vi "Dashboard Main - Copy.vi"() -> ()   [LabVIEW 2011]
panel:
  out "TARGET AQUIRED":bool
  out "FAILSAFE!":bool
  out "Right":T1(plugin-control)
  out "Left":T1(plugin-control)
  in  "Tab Control":enum32{"Operator", "Diagnotics"}(tab)
  out "Shooter RPM":dbl(knob) scale=0.0..4000.0
  out "Limit Right":bool
  out "Limit Left":bool
  out "Turret Postition":dbl(knob) scale=240.0..-60.0
  out "Home":bool
  out "1":bool
  out "2":bool
  out "3":bool
  out "Bridge Balance":bool
  out "Intake Reverse":bool
  out "Intake Foward":bool
  out "High Gear":bool
  out "Low Gear":bool
  out "Robot IP Address":string
  out "Battery Voltage":dbl(slide) scale=8.0..14.0
  out "Distance From Target":dbl
  in  "Distance adjust":dbl
  in  "Left camera adjust":dbl
  in  "Right camera adjust":dbl
  out "Turret Enc":dbl
  out "Compass":dbl(knob) scale=0.0..-180.0
  out "Shooter Ready":bool
  out "Right Drive":dbl
  out "Left Drive":dbl
  out "Gyro":dbl(knob) scale=-180.0..180.0
  out "Primed":bool
  out "Upper Belt":bool
  out "Lower Belt":bool
  out "Entrance":bool
  in  "Video Enable":bool=TRUE
  in  "LED Color":enum32{"RED", "BLUE", "PURPLE"}(radio)
  out "FIRE!":bool
  out "Dashboard Datatype Warning":string="Warning: The Dashboard Datatype used by the robot project and this dashboard do not match.\nSee diagram for more details."
  # "Ball Count"
  # "Communications"
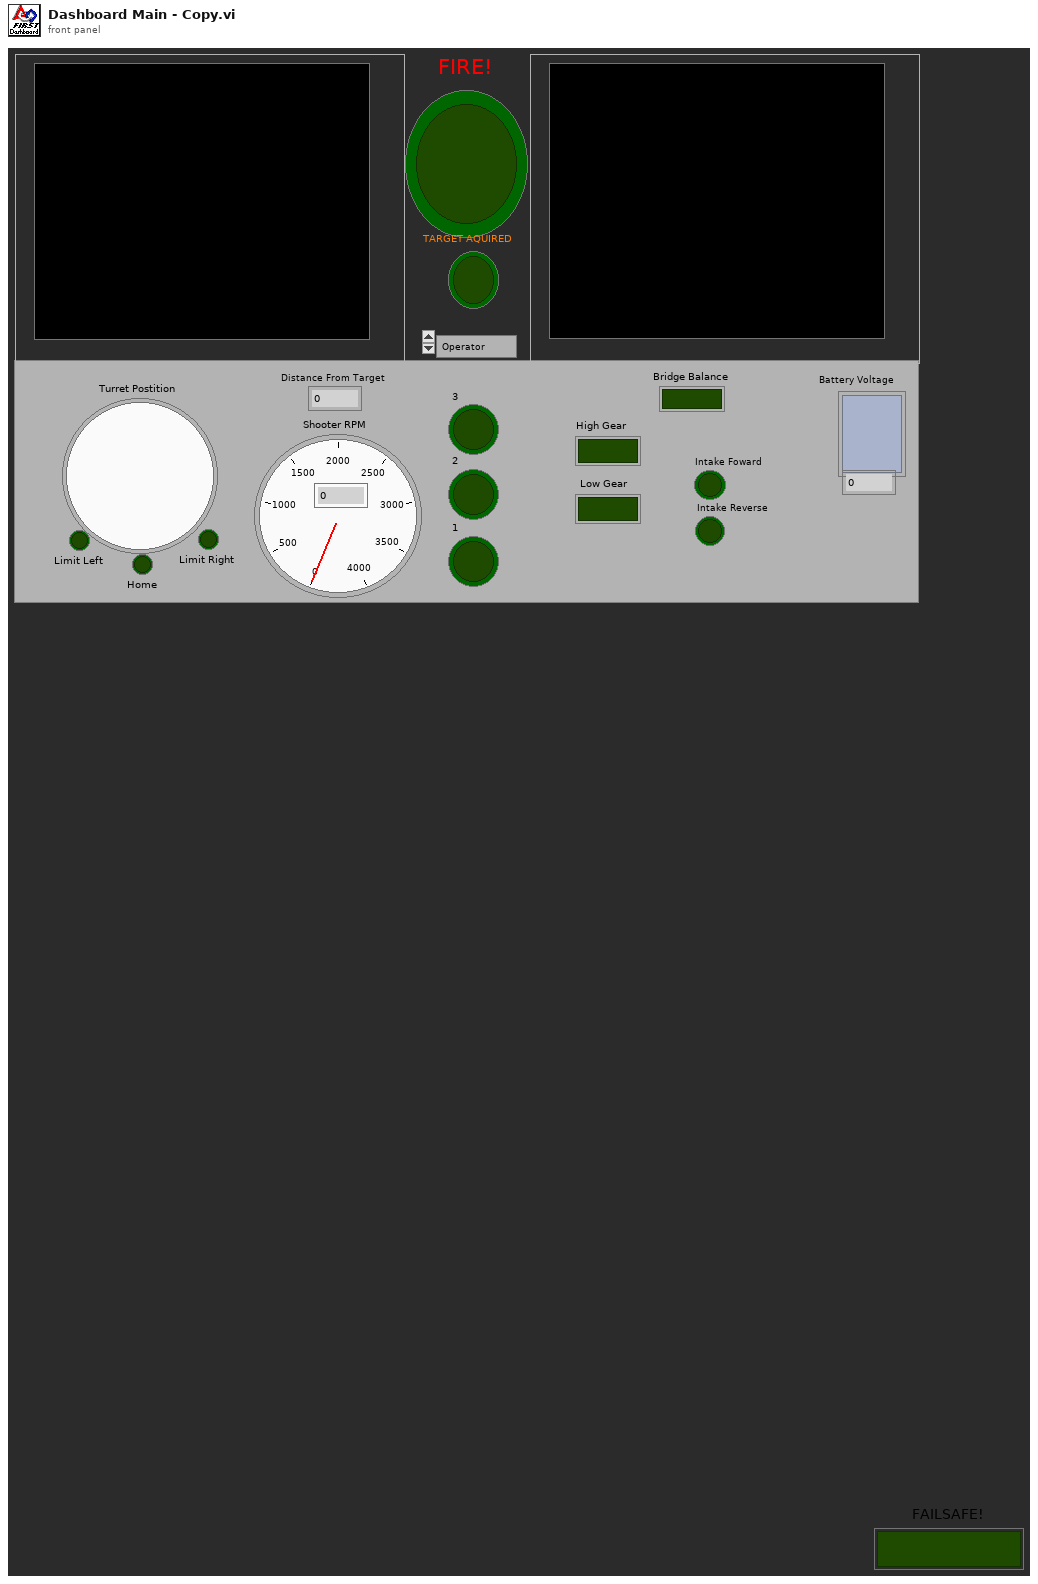
[diagram p1: front panel]
types:
  T1 = typedef "IMAQ Image.ctl" = refnum<image>
  T2 = cluster{"Home":bool, "Distance From Target":dbl, "Ball Count":dbl, "Gear":u16, "Shooter RMP":dbl, "Target Acuired":bool, "FIRE":bool, "Intake Motor direction":dbl, "FailSafe":bool}
  T3 = cluster{"Distance From Target":dbl, "Bridge Balance":bool, "Entrance":bool, "Lower Belt":bool, "Upper Belt":bool, "Primed":bool, "Turret Postition":dbl, "Gyro":dbl, "Left Drive":dbl, "Right Drive":dbl, "Home":bool, "Limit Left":dbl, "Limit Right":dbl, "Shooter Ready":bool, "Compass":dbl, "Turret Enc":dbl, "Ball Count":dbl, "Intake":dbl}
  T4 = typedef "Image Type" = u32
  T5 = cluster{"Competition mode":bool, "Robot Link":bool, "Autonomous":bool, "Enabled":bool, "E-Stop":bool}
  T6 = cluster{"Boolean array[0]":bool, "Boolean array[1]":bool, "Boolean array[2]":bool, "Boolean array[3]":bool, "Boolean array[4]":bool, "Boolean array[5]":bool, "Boolean array[6]":bool, "Boolean array[7]":bool, "Boolean array[8]":bool}
  T7 = typedef "LVRectTypeDef.ctl" = cluster{"left":i16, "top":i16, "right":i16, "bottom":i16}
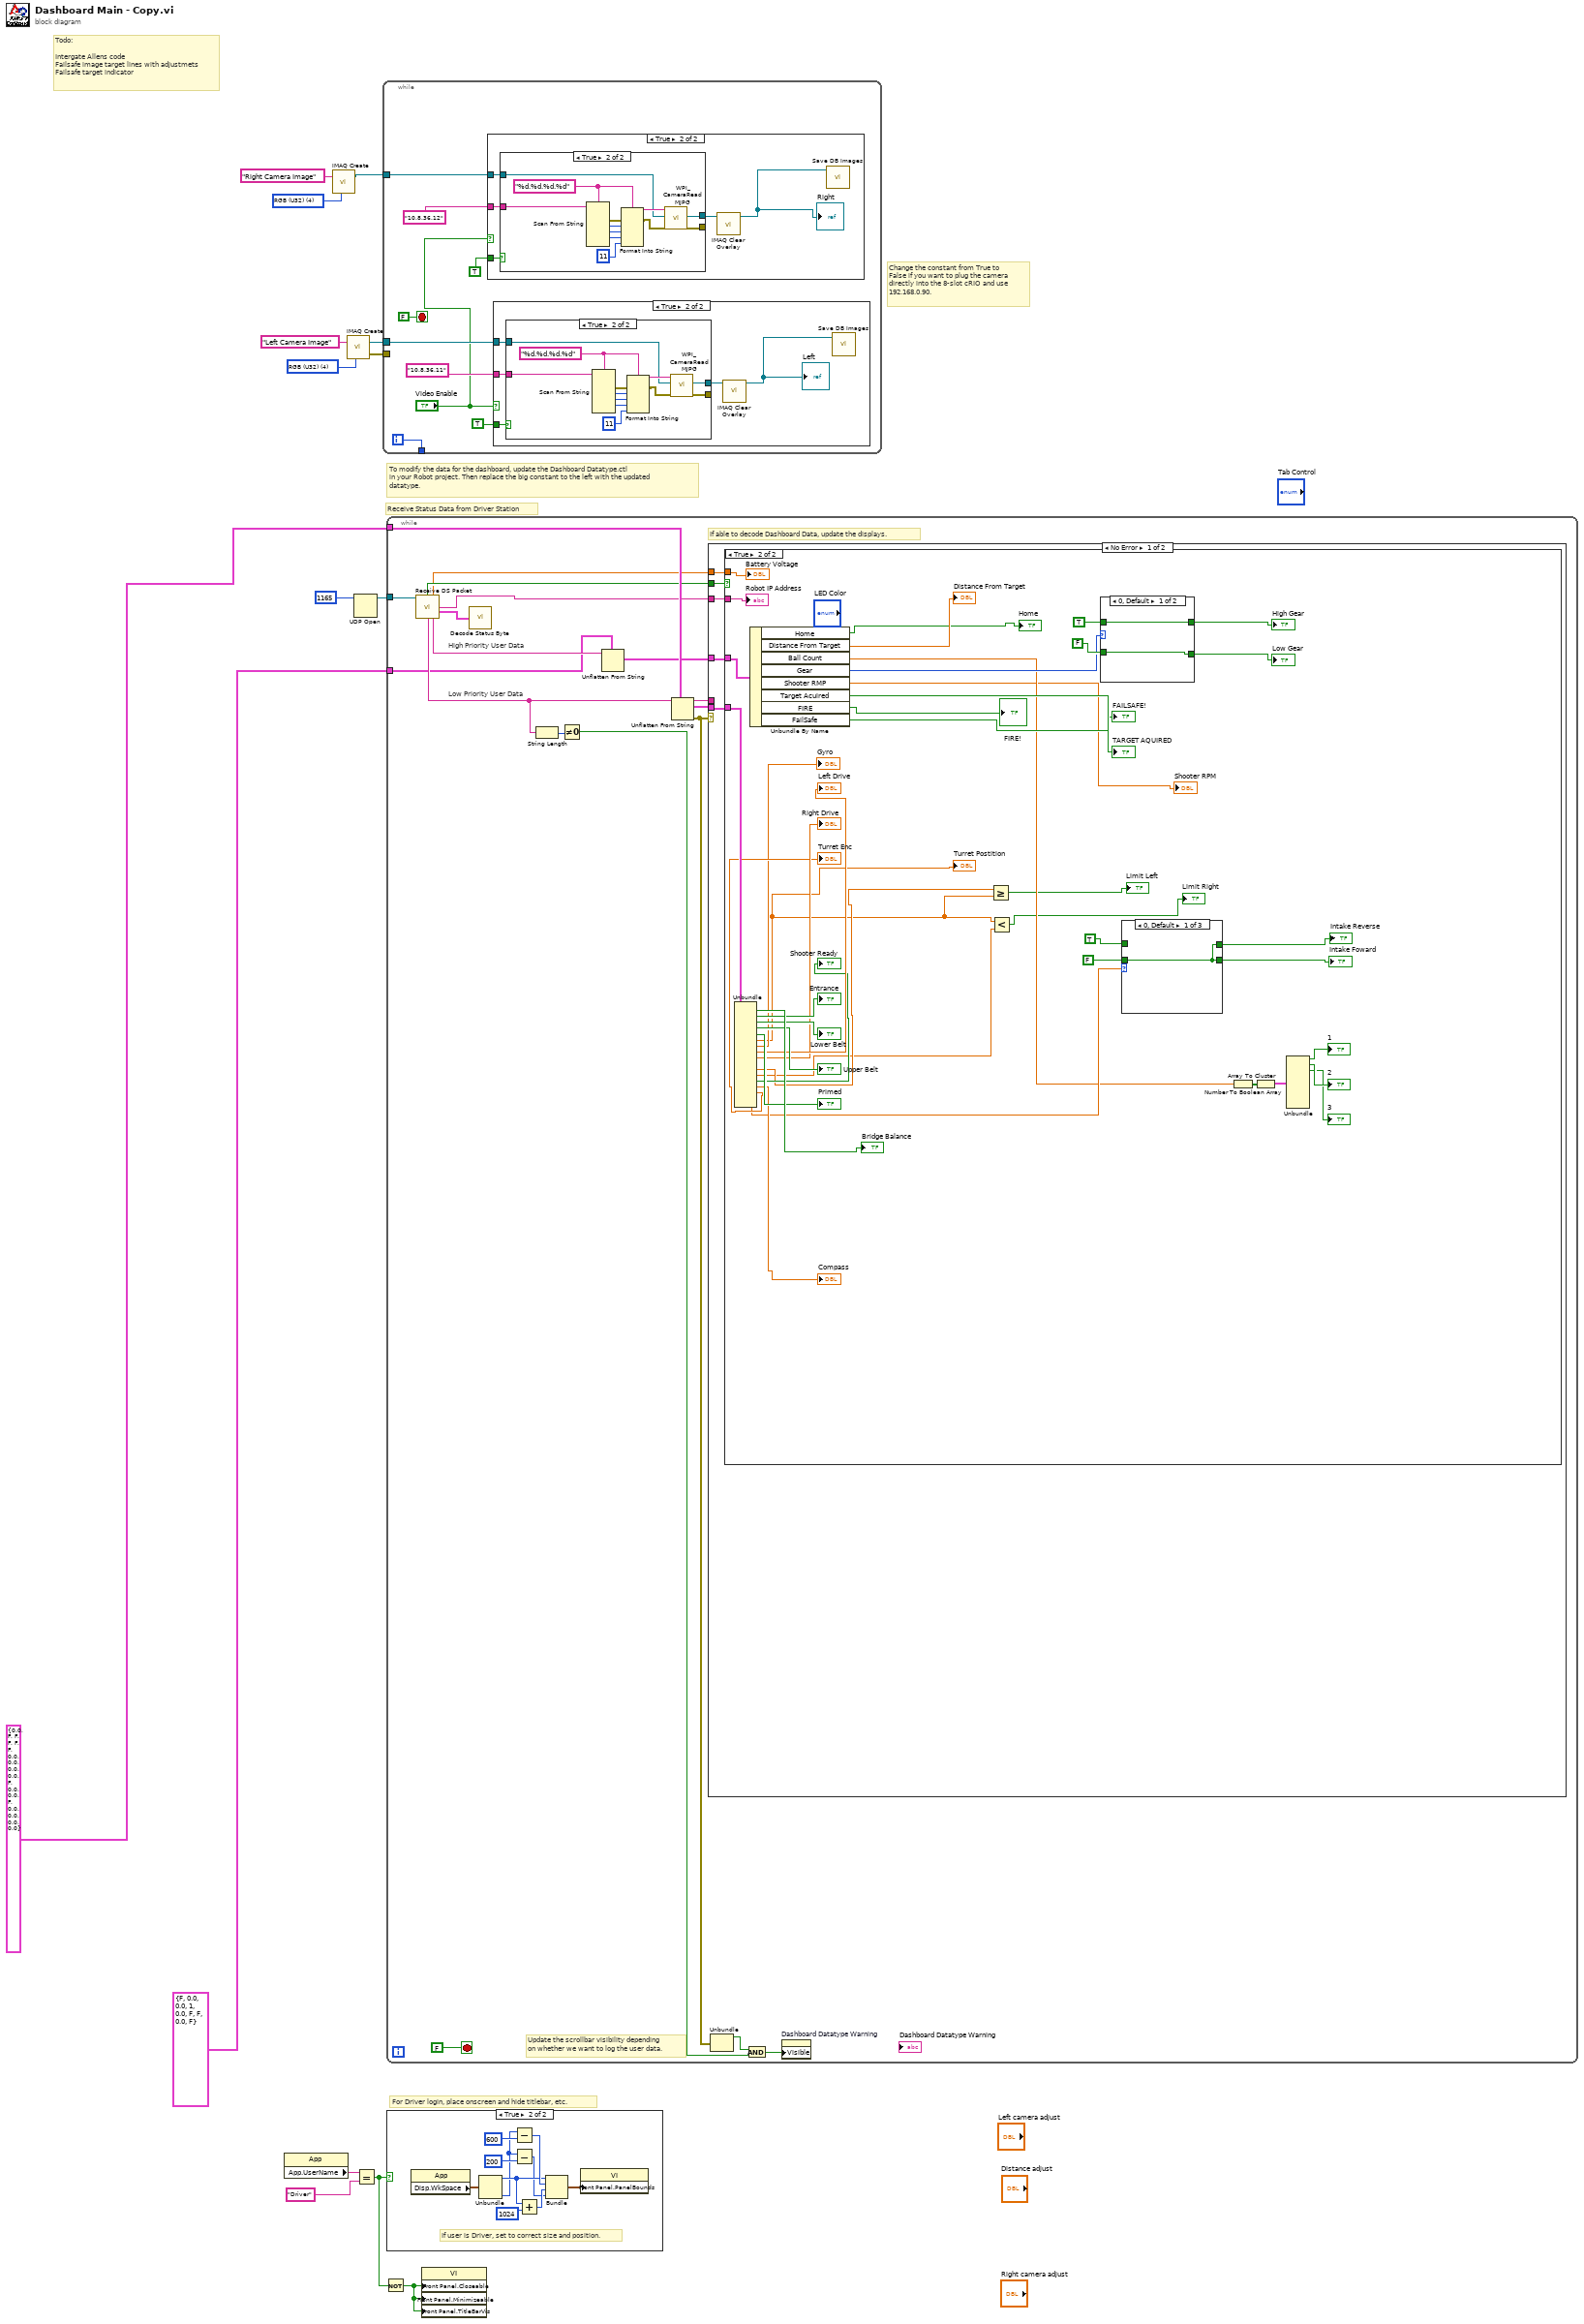
[diagram p0: block diagram]
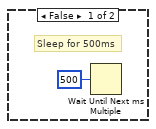
[diagram p8: hidden frame]
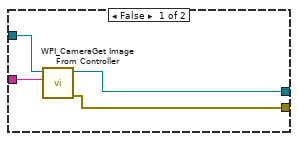
[diagram p9: hidden frame]
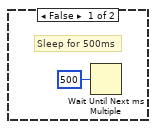
[diagram p10: hidden frame]
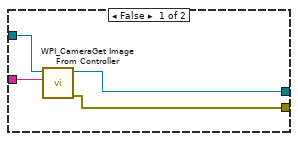
[diagram p11: hidden frame]
diagram:
  w5 = T4 4 items=["Grayscale (U8)", "Grayscale (I16)", "Grayscale (SGL)", "Complex (CSG)", "RGB (U32)", "HSL (U32)", "RGB (U64)"] ("Image Type")
  w13 = T4 4 items=["Grayscale (U8)", "Grayscale (I16)", "Grayscale (SGL)", "Complex (CSG)", "RGB (U32)", "HSL (U32)", "RGB (U64)"] ("Image Type")
  # "Todo: \n\nIntergate Allens code\nFailsafe image target lines with adjustmets\nFailsafe target indicator"
  # "Change the constant from True to\nFalse if you want to plug the camera\ndirectly into the 8-slot cRIO and use\n192.168.0.90."
  # "For Driver login, place onscreen and hide titlebar, etc."
  # "To modify the data for the dashboard, update the Dashboard Datatype.ctl\nin your Robot project. Then replace the big constant to the left with the updated\ndatatype."
  # "Receive Status Data from Driver Station"
  n1 = property class="App"() -> ("App.UserName"=w8:string)  [unwired: 2 in, 2 out]
  n2 = call "IMAQ Create"("Image Name"="Right Camera Image", "Image Type"=w5) -> ("New Image"=w3:T1)  [unwired: 2 in, 2 out]
  n3 = call "IMAQ Create"("Image Name"="Left Camera Image", "Image Type"=w13) -> ("New Image"=w11:T1, "error out"=w10:errorcluster)  [unwired: 2 in, 1 out]
  n4 = UDP Open(11:u16 1165 ("port")) -> (port=w14:refnum<k16>)  [unwired: 2 in, 4 out]
  n5 = Equal?(x=w8, y="Driver") -> (x = y?=w7:bool)
  n6 = while {
    tunnel: w11 -> [w23]
    tunnel: w10 -> [_]
    tunnel: [w21] -> _
    tunnel: w3 -> [w17]
    i -> [w21]
    stop <- FALSE stop-if-true
    n7 = case shown="True" "Video Enable" {
      tunnel: "10.8.36.12" ("input string") -> [_ w30]
      tunnel: w17 -> [_ w29]
      tunnel: TRUE -> [_ w27]
      frame False {
        # "Sleep for 500ms"
        n8 = Wait Until Next ms Multiple(millisecond multiple=u32 500) -> ()  [unwired: 1 out]
      }
      frame True {
        n9 = case shown="True" w27 {
          tunnel: w29 -> [w33 w40]
          tunnel: [w31 w38] -> _
          tunnel: [w32 w39] -> w28
          tunnel: w30 -> [w34 w43]
          frame False {
            n10 = call <vilib>:"WPI_CameraGet Image From Controller.vi"("Controller Address"=w34, "Image"=w33) -> ("error out"=w31:errorcluster, "Image Out"=w32:T1)  [unwired: 2 in, 6 out]
          }
          frame True {
            w35 = "%d.%d.%d.%d" ("format string")
            n11 = Scan From String(format string=w35, input string=w43) -> (error out=w42:errorcluster, output 1=w44:i32, output 2=w45:i32, output 3=w46:i32)  [unwired: 2 in, 7 out]
            n12 = Format Into String(format string=w35, error in=w42, w44, w45, w46, 11 ("IP Suffix:")) -> (resulting string=w41:string, error out=w37:errorcluster)  [unwired: 1 in]
            n13 = call <vilib>:"WPI_CameraRead MJPG.vi"("error in"=w37, "Image"=w40, "address"=w41) -> ("error out"=w38:errorcluster, "Image Out"=w39:T1)  [unwired: 7 in]
          }
        }
        n14 = call "IMAQ Clear Overlay"("Image"=w28) -> ("Image Out"=w26:T1)  [unwired: 2 in, 8 out]
        "Right" <- w26
        n15 = call "Save DB Images.vi"("Image"=w26) -> ()  [unwired: 2 in, 1 out]
      }
    }
    n16 = case shown="True" "Video Enable" {
      tunnel: "10.8.36.11" ("input string") -> [_ w52]
      tunnel: w23 -> [_ w51]
      tunnel: TRUE -> [_ w49]
      frame False {
        # "Sleep for 500ms"
        n17 = Wait Until Next ms Multiple(millisecond multiple=u32 500) -> ()  [unwired: 1 out]
      }
      frame True {
        n18 = case shown="True" w49 {
          tunnel: w51 -> [w55 w62]
          tunnel: [w53 w60] -> _
          tunnel: [w54 w61] -> w50
          tunnel: w52 -> [w56 w65]
          frame False {
            n19 = call <vilib>:"WPI_CameraGet Image From Controller.vi"("Controller Address"=w56, "Image"=w55) -> ("error out"=w53:errorcluster, "Image Out"=w54:T1)  [unwired: 2 in, 6 out]
          }
          frame True {
            w57 = "%d.%d.%d.%d" ("format string")
            n20 = Scan From String(format string=w57, input string=w65) -> (error out=w64:errorcluster, output 1=w66:i32, output 2=w67:i32, output 3=w68:i32)  [unwired: 2 in, 7 out]
            n21 = Format Into String(format string=w57, error in=w64, w66, w67, w68, 11 ("IP Suffix:")) -> (resulting string=w63:string, error out=w59:errorcluster)  [unwired: 1 in]
            n22 = call <vilib>:"WPI_CameraRead MJPG.vi"("error in"=w59, "Image"=w62, "address"=w63) -> ("error out"=w60:errorcluster, "Image Out"=w61:T1)  [unwired: 7 in]
          }
        }
        n23 = call "IMAQ Clear Overlay"("Image"=w50) -> ("Image Out"=w48:T1)  [unwired: 2 in, 8 out]
        "Left" <- w48
        n24 = call "Save DB Images.vi"("Image"=w48) -> ()  [unwired: 2 in, 1 out]
      }
    }
  }
  n25 = Not(x=w7) -> (.not. x?=w6:bool)
  n26 = while {
    tunnel: w14 -> [w84]
    tunnel: T3 {"Distance From Target"=0.0, "Bridge Balance"=FALSE, "Entrance"=FALSE, "Lower Belt"=FALSE, "Upper Belt"=FALSE, "Primed"=FALSE, "Turret Postition"=0.0, "Gyro"=0.0, "Left Drive"=0.0, "Right Drive"=0.0, "Home"=FALSE, "Limit Left"=0.0, "Limit Right"=0.0, "Shooter Ready"=FALSE, "Compass"=0.0, "Turret Enc"=0.0, "Ball Count"=0.0, "Intake"=0.0} ("Dashboard Data") -> [w83]
    tunnel: T2 {"Home"=FALSE, "Distance From Target"=0.0, "Ball Count"=0.0, "Gear"=1, "Shooter RMP"=0.0, "Target Acuired"=FALSE, "FIRE"=FALSE, "Intake Motor direction"=0.0, "FailSafe"=FALSE} ("HiPri") -> [w70]
    stop <- FALSE stop-if-true
    # "High Priority User Data"
    # "Low Priority User Data"
    # "Update the scrollbar visibility depending\non whether we want to log the user data."
    # "If able to decode Dashboard Data, update the displays."
    n27 = call "Receive DS Packet.vi"("Recv Socket"=w84) -> ("New Dashboard Data"=w80:bool, "Battery"=w72:sgl, "Robot IP Address"=w71:string, "Status"=w85:T5, "Low Priority User Data"=w74:string, "High Priority User Data"=w73:string)  [unwired: 1 in, 8 out]
    n28 = call "Decode Status Byte.vi"("Status Byte"=w85) -> ()  [unwired: 2 out]
    n29 = String Length(string=w74) -> (length=w75:i32)
    n30 = Not Equal To 0?(x=w75) -> (x != 0?=w78:bool)
    n31 = Unflatten From String(type=w70, binary string=w73) -> (value=w69:T2)  [unwired: 1 in, 4 out]
    n32 = Unflatten From String(type=w83, binary string=w74) -> (rest of the binary string=w76:string, value=w82:T3, error out=w81:errorcluster)  [unwired: 1 in, 2 out]
    n33 = case shown="No Error" w81 {
      tunnel: w82 -> [w91 _]
      tunnel: w80 -> [w90 _]
      tunnel: w76 -> [_ _]
      tunnel: w72 -> [w89 _]
      tunnel: w71 -> [w88 _]
      tunnel: w69 -> [w87 _]
      frame No Error {
        n34 = case shown="True" w90 {
          tunnel: w91 -> [_ w133]
          tunnel: w89 -> [_ w132]
          tunnel: w88 -> [_ w131]
          tunnel: w87 -> [_ w103]
          frame False {
            # "Don't update if the robot hasn't sent new data"
          }
          frame True {
            n35 = Unbundle(w133) -> ("Bridge Balance"=→"Bridge Balance":bool, "Entrance"=→"Entrance":bool, "Lower Belt"=→"Lower Belt":bool, "Upper Belt"=→"Upper Belt":bool, "Primed"=→"Primed":bool, "Turret Postition"=w92:dbl, "Gyro"=→"Gyro":dbl, "Left Drive"=→"Left Drive":dbl, "Right Drive"=→"Right Drive":dbl, "Limit Left"=w105:dbl, "Limit Right"=w104:dbl, "Shooter Ready"=→"Shooter Ready":bool, "Compass"=→"Compass":dbl, "Turret Enc"=→"Turret Enc":dbl, "Intake"=w107:dbl)  [unwired: 3 out]
            "Turret Postition" <- w92
            n36 = Unbundle By Name(w103) -> ("Home"=→"Home":bool, "Distance From Target"=→"Distance From Target":dbl, "Ball Count"=w98:dbl, "Gear"=w101:u16, "Shooter RMP"=→"Shooter RPM":dbl, "Target Acuired"=→"TARGET AQUIRED":bool, "FIRE"=→"FIRE!":bool, "FailSafe"=→"FAILSAFE!":bool)
            n37 = Greater Or Equal?(x=w105, y=w92) -> (x >= y?=→"Limit Left":bool)
            n38 = Less?(x=w92, y=w104) -> (x < y?=→"Limit Right":bool)
            n39 = case shown="0, Default" w101 {
              tunnel: TRUE -> [w140 w142]
              tunnel: [w140 w141] -> w124
              tunnel: [w139 w142] -> w123
              tunnel: FALSE -> [w139 w141]
              frame 0, Default {
              }
              frame 1 {
              }
            }
            "Low Gear" <- w123
            "High Gear" <- w124
            n40 = case shown="0, Default" w107 {
              tunnel: [w134 w136 w138] -> w120
              tunnel: FALSE -> [w134 w135 w137]
              tunnel: [w134 w135 w137] -> w119
              tunnel: TRUE -> [_ w136 w138]
              frame 0, Default {
              }
              frame 1 {
              }
              frame -1 {
              }
            }
            "Intake Foward" <- w120
            "Intake Reverse" <- w119
            n41 = Number To Boolean Array(number=w98) -> (Boolean array=w130:bool[])
            n42 = Array To Cluster(array=w130) -> (cluster=w129:T6)
            n43 = Unbundle(w129) -> ("Boolean array[0]"=→"1":bool, "Boolean array[1]"=→"2":bool, "Boolean array[2]"=→"3":bool)  [unwired: 6 out]
            "Battery Voltage" <- w132
            "Robot IP Address" <- w131
          }
        }
      }
      frame Error {
        # "Your datatypes don't match. The Dashboard Datatype.ctl in your Robot project\nand the big constant to the left of the loop need to match."
      }
    }
    n44 = Unbundle(w81) -> ("status"=w77:bool)  [unwired: 2 out]
    n45 = And(x=w77, y=w78) -> (x .and. y?=w79:bool)
    n46 = property on="Dashboard Datatype Warning" class="Str"("Visible"=w79) -> ()  [unwired: 2 in, 2 out]
  }
  n47 = case shown="True" w7 {
    frame False {
    }
    frame True {
      # "If user is Driver, set to correct size and position."
      n48 = property class="App"() -> ("Disp.WkSpace"=w152:T7)  [unwired: 2 in, 2 out]
      n49 = Unbundle(w152) -> ("left"=w147:i16, "bottom"=w143:i16)  [unwired: 2 out]
      n50 = Subtract(x=w143, y=600) -> (x-y=w149:i32)
      n51 = Subtract(x=w143, y=200) -> (x-y=w144:i32)
      n52 = Add(x=w147, y=1024) -> (x+y=w148:i32)
      n53 = Bundle("left"=w147, w149, w148, w144) -> (w151:cluster{"left":i16, i32, i32, i32})  [unwired: 1 out]
      n54 = property class="VI"("Front Panel.PanelBounds"=w151) -> ()  [unwired: 2 in, 2 out]
    }
  }
  n55 = property class="VI"("Front Panel.Closeable"=w6, "Front Panel.Minimizeable"=w6, "Front Panel.TitleBarVis"=w6) -> ()  [unwired: 2 in, 2 out]
